vi "SimpleGit_Item_OnCommand.vi"(10 "Command ID":string, 11 "Object":T1) -> ()   [LabVIEW 2017]
uses:
  <resource>/Framework/Providers/API/ItemRef.ctl
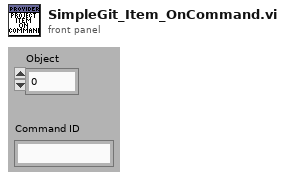
[diagram p1: front panel]
types:
  T1 = typedef "ItemRef.ctl" = u64
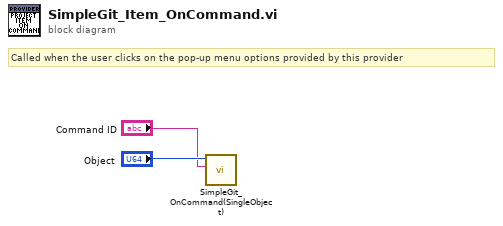
[diagram p0: block diagram]
diagram:
  # "Called when the user clicks on the pop-up menu options provided by this provider"
  n1 = call "SimpleGit_OnCommand(SingleObject).vi"("Command ID"="Command ID", "Object"="Object") -> ()  [unwired: 10 in]
